vi "PXI-Set AO Gains OTF.vi"(8 "error in (no error)":errorcluster) -> (0 "error out":errorcluster)   [LabVIEW 2020]
uses:
  PXI Globals.vi
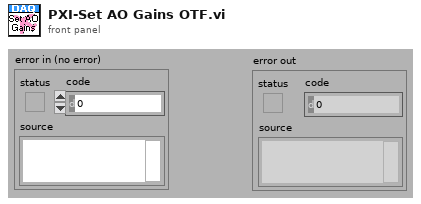
[diagram p1: front panel]
types:
  T1 = enum16{"Init", "Write", "Read", "Latch setup", "Compute comp."}
  T2 = typedef "Task Struct.ctl" = cluster{"Task name":string, "Task":refnum<k21>, "Dual-channel task?":bool, "Regenerate?":bool, "Clear?":bool}
  T3 = enum16{"Init", "Write", "Read", "Latch setup", "Compute comp.", "Read 1 Channel"}
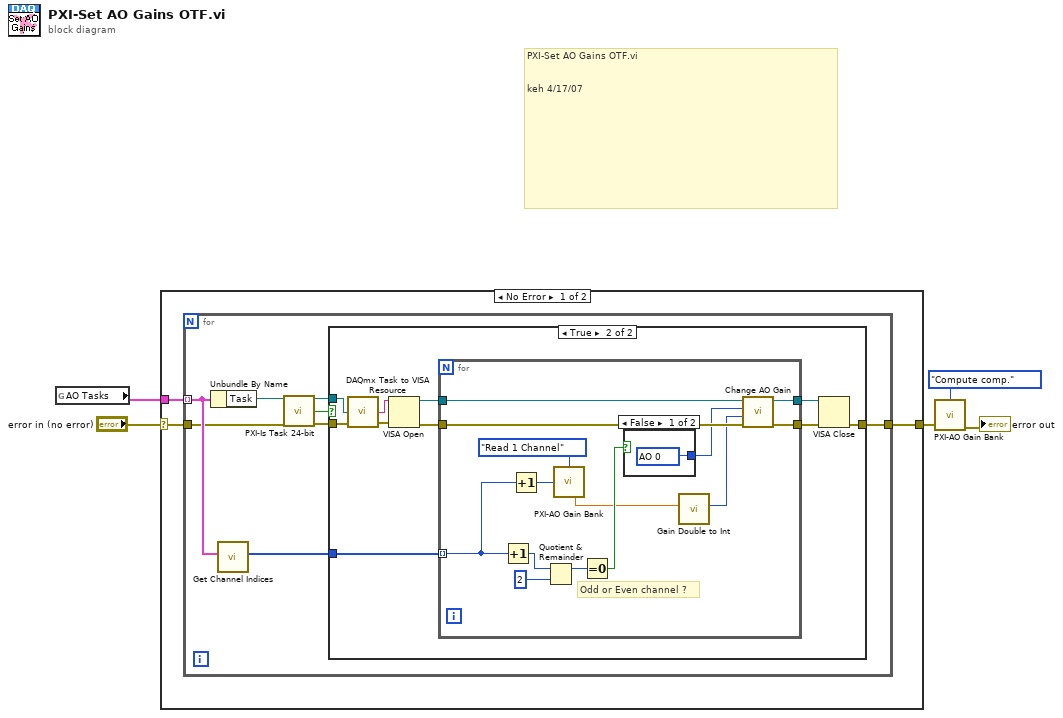
[diagram p0: block diagram]
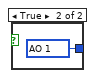
[diagram p3: hidden frame]
diagram:
  # "PXI-Set AO Gains OTF.vi\n\n\nkeh 4/17/07"
  n1 = global read "PXI Globals.vi" "AO Tasks"() -> (w4:T2[])
  n2 = case shown="No Error" "error in (no error)" {
    selector: "error in (no error)" -> [w7 w44]
    tunnel: [w6 w44] -> w3
    tunnel: w4 -> [w8 _]
    frame No Error {
      n3 = for {
        tunnel: w8 -> [w16] mode=indexing
        tunnel: w7 -> [w10]
        tunnel: [w14] -> w6
        n4 = Unbundle By Name(w16) -> ("Task"=w13:refnum<k21>)
        n5 = call "Get Channel Indices.vi"("Task Structure"=w16) -> ("Channel Indices"=w15:i32[])  [unwired: 10 in]
        n6 = call "PXI-Is Task 24-bit.vi"("task"=w13, "error in (no error)"=w10) -> ("task out"=w11:refnum<k21>, "is 24bit?"=w9:bool, "error out"=w12:errorcluster)  [unwired: 8 in, 3 out]
        n7 = case shown="True" w9 {
          tunnel: w15 -> [_ w27]
          tunnel: [w17 w26] -> w14
          tunnel: w12 -> [w17 w18]
          tunnel: w11 -> [_ w19]
          frame False {
          }
          frame True {
            n8 = call "DAQmx Task to VISA Resource.vi"("error in (no error)"=w18, "task out"=w19) -> ("error out"=w20:errorcluster, "VISAName"=w21:string)  [unwired: 2 in]
            n9 = VISA Open(error in (no error)=w20, VISA resource name=w21) -> (VISA resource name=w25:refnum<visa-resource-name>, error out=w23:errorcluster)  [unwired: 3 in]
            n10 = for {
              tunnel: w23 -> [w41]
              tunnel: [w40] -> w22
              tunnel: w27 -> [w39] mode=indexing
              tunnel: w25 -> [w38]
              tunnel: [w37] -> w24
              # "Odd or Even channel ?"
              n11 = Increment(x=w39) -> (x+1=w32:i32)
              n12 = Increment(x=w39) -> (x+1=w28:i32)
              n13 = Quotient & Remainder(x=w32, y=2) -> (x-y*floor(x/y)=w33:i32)  [unwired: 1 out]
              n14 = call "PXI-AO Gain Bank.vi"("Action"=T3."Read 1 Channel", "AO channel"=w28) -> ("Gain 1 channel"=w30:dbl)  [unwired: 8 in, 5 out]
              n15 = Equal To 0?(x=w33) -> (x = 0?=w31:bool)
              n16 = case shown="False" w31 {
                tunnel: [w42 w43] -> w35
                frame False {
                  w42 = u16 1536 items=["AO 0"=1536, "AO 1"=1540] ("AO Channel")
                }
                frame True {
                  w43 = u16 1540 items=["AO 0"=1536, "AO 1"=1540] ("AO Channel")
                }
              }
              n17 = call "Gain Double to Int.vi"("Gain Double"=w30) -> ("Gain Setting"=w36:u16)  [unwired: 10 in]
              n18 = call "Change AO Gain.vi"("error in"=w41, "Gain Setting"=w36, "AO Channel"=w35, "VISA resource name 2"=w38) -> ("error out"=w40:errorcluster, "VISA resource name"=w37:refnum<visa-resource-name>)  [unwired: 4 in]
            }
            n19 = VISA Close(VISA resource name=w24, error in (no error)=w22) -> (error out=w26:errorcluster)
          }
        }
      }
    }
    frame Error {
    }
  }
  n20 = call "PXI-AO Gain Bank.vi"("Action"=T1."Compute comp.", "error in (no error)"=w3) -> ("error out"=→"error out":errorcluster)  [unwired: 8 in, 5 out]
